vi "Spherical Bessel Function yn.vi"(2 "n":i32, 3 "x":dbl format="%.2f") -> (1 "yn(x)":dbl format="%.2f")   [LabVIEW 2010, in "NI_Gmath.lvlib"]
doc: "Calculates the spherical Bessel function of the second kind."
uses:
  NI_Gmath.lvlib
  lvanlys.dll
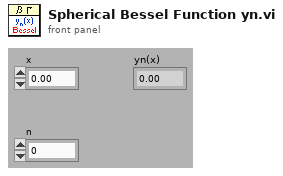
[diagram p1: front panel]
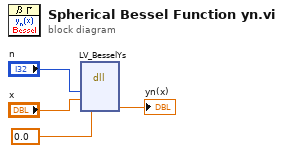
[diagram p0: block diagram]
diagram:
  n1 = dll-call lib="C:/Program Files/National Instruments/LabVIEW 2010/resource/lvanlys.*" fn="LV_BesselYs"("n"="n", "x"="x", "yn(x)"=0.0 ("Jr")) -> ("yn(x)"=→"yn(x)":dbl)  [unwired: 6 in, 2 out]
